vi "Read Attributes.vi"(11 "Image Msg":refnum<class "Image Msg.lvclass">) -> (2 "Payload":cluster{"Image":T1})   [LabVIEW 2016, in "Image Acquisition.lvlib" / "Image Msg.lvclass"]
uses:
  Image Msg.lvclass
  <vilib>/vision/Image Controls.llb/IMAQ Image.ctl
  Image Msg.lvclass/Image Msg.ctl
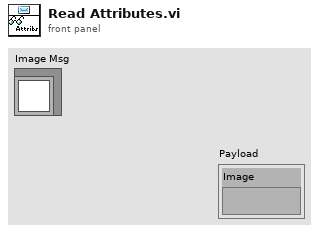
[diagram p1: front panel]
types:
  T1 = typedef "IMAQ Image.ctl" = refnum<image>
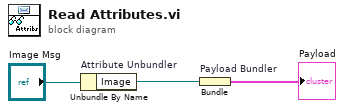
[diagram p0: block diagram]
diagram:
  n1 = Unbundle By Name "Attribute Unbundler"("Image Msg") -> ("Image"=w1:T1)
  n2 = Bundle "Payload Bundler"("Image"=w1) -> (→"Payload":cluster{"Image":T1})  [unwired: 1 in]
